vi "FOTOS.vi"() -> ()   [LabVIEW 2017]
panel:
  in  "Muestreo B (sec)":i32=60
  in  "Intervalo B (min)":i32=60
  in  "Intervalo A (min)":i32=1
  in  "Muestreo A (sec)":i32=1
  in  "run minimized? (F)":bool caption="Checkbox"
  out "Command line":string
  in  "wait until completion? (T)":bool caption="Checkbox"
  out "standard output":string
  in  "Power On Button":bool
  out "Numeric":i32
  in  "Start webcam":bool
  # "Configurar y arrancar webcam"
  # "asslcdms Feb2023 LV17"
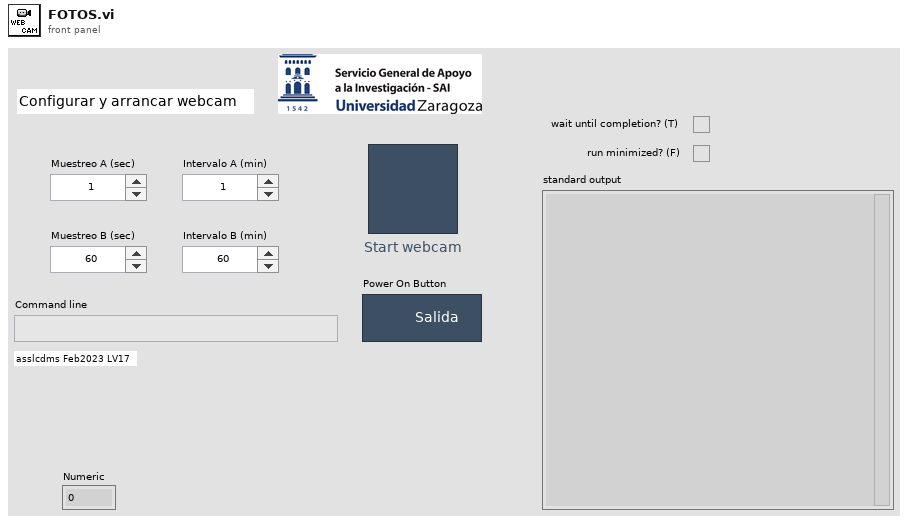
[diagram p1: front panel]
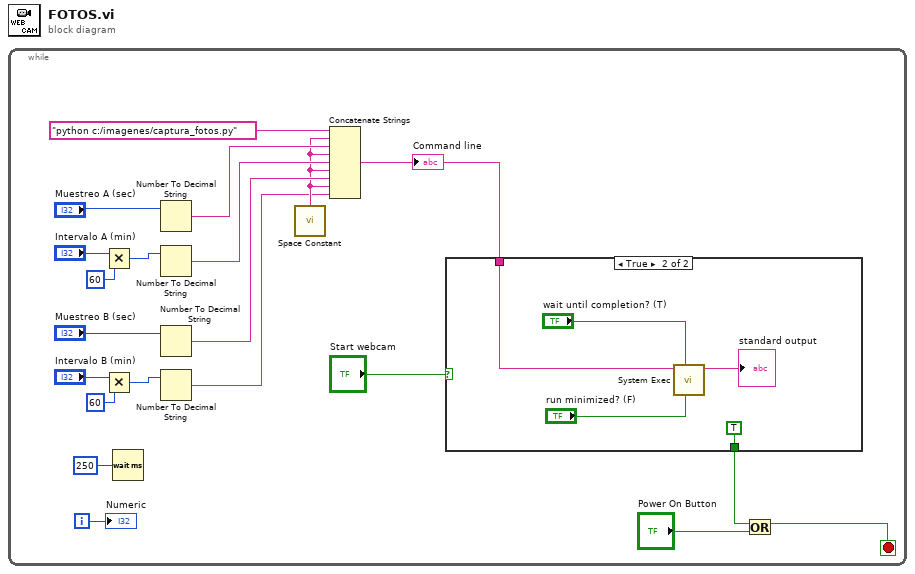
[diagram p0: block diagram]
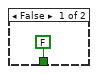
[diagram p2: hidden frame]
diagram:
  n1 = while {
    i -> [w21]
    stop <- w5 stop-if-true
    n2 = Multiply(x="Intervalo A (min)", y=60) -> (x*y=w8:i32)
    n3 = Multiply(x="Intervalo B (min)", y=60) -> (x*y=w7:i32)
    n4 = Wait (ms)(milliseconds to wait=u32 250) -> ()  [unwired: 1 out]
    n5 = Number To Decimal String(number="Muestreo A (sec)") -> (decimal integer string=w16:string)  [unwired: 1 in]
    n6 = Number To Decimal String(number=w8) -> (decimal integer string=w15:string)  [unwired: 1 in]
    n7 = Number To Decimal String(number="Muestreo B (sec)") -> (decimal integer string=w14:string)  [unwired: 1 in]
    n8 = Number To Decimal String(number=w7) -> (decimal integer string=w12:string)  [unwired: 1 in]
    n9 = call <vilib>:"Space Constant.vi"() -> ("String"=w13:string)
    n10 = Concatenate Strings("python c:/imagenes/captura_fotos.py" ("Command line"), w13, w16, w13, w15, w13, w14, w13, w12) -> (w11:string)
    "Command line" <- w11
    n11 = case shown="True" "Start webcam" {
      tunnel: w11 -> [_ w24]
      tunnel: [FALSE TRUE] -> w3
      frame False {
      }
      frame True {
        n12 = call <vilib>:"System Exec.vi"("run minimized? (F)"="run minimized? (F)", "wait until completion? (T)"="wait until completion? (T)", "command line"=w24) -> ("standard output"=→"standard output":string)  [unwired: 5 in, 3 out]
      }
    }
    n13 = Or(x=w3, y="Power On Button") -> (x .or. y?=w5:bool)
    "Numeric" <- w21
  }
